vi "Z complex to real imag.vi"(8 "Error In":errorcluster, 9 "Z (cplx)":T2 {"Z" format="%#_4g"}) -> (0 "Error Out":errorcluster, 1 "imag Z":T1, 2 "real Z":T1)   [LabVIEW 2016]
uses:
  Trace (dbl).ctl
  Trace (cplx).ctl
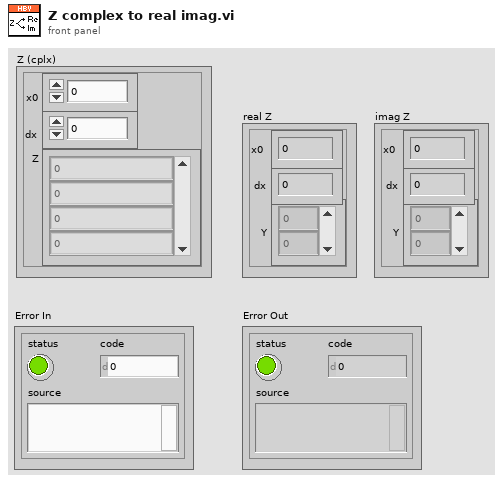
[diagram p1: front panel]
types:
  T1 = typedef "Trace (dbl).ctl" = cluster{"x0 ":dbl, "dx":dbl, "Y":dbl[]}
  T2 = typedef "Trace (cplx).ctl" = cluster{"x0":dbl, "dx":dbl, "Z":cdb[]}
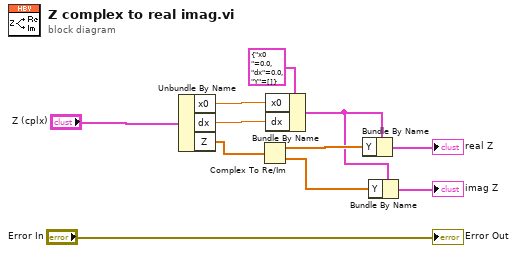
[diagram p0: block diagram]
diagram:
  n1 = Unbundle By Name("Z (cplx)") -> ("x0"=w6:dbl, "dx"=w5:dbl, "Z"=w2:cdb[])
  n2 = Complex To Re/Im(x + iy=w2) -> (x=w9:dbl[], y=w7:dbl[])
  n3 = Bundle By Name(cluster=T1 {"x0 "=0.0, "dx"=0.0, "Y"=[]} ("Spectrum"), "x0"=w6, "dx"=w5) -> (w1:T1)
  n4 = Bundle By Name(cluster=w1, "Y"=w9) -> (→"real Z":T1)
  n5 = Bundle By Name(cluster=w1, "Y"=w7) -> (→"imag Z":T1)
  "Error Out" <- "Error In"
